vi "NanotecSMCPDDriver.self test.vi"(0 "VISA resource name":refnum<visa-resource-name>, 1 "contollerID":i32=-1, 5 "error in (no error)":errorcluster) -> (14 "VISA resource name out":refnum<visa-resource-name>, 15 "contollerID out":i32=-1, 17 "Self-Test Result Code":i32, 18 "Self-Test Result Message":string, 19 "error out":errorcluster)   [LabVIEW 2014, in "NanotecSMCPDDriver.lvlib"]
doc: "Runs the instrument's self-test routine and returns the test results."
uses:
  NanotecSMCPDDriver.lvlib
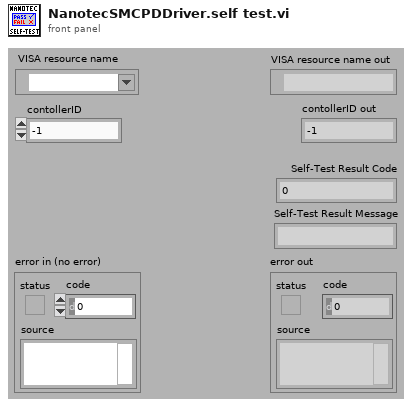
[diagram p1: front panel]
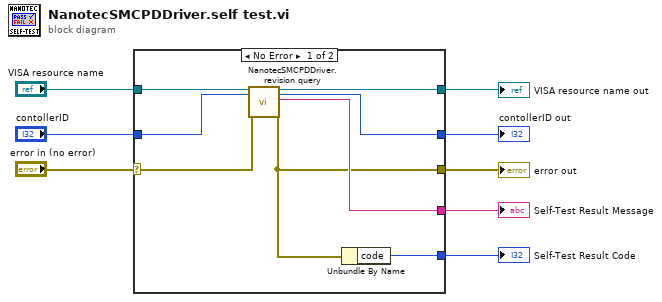
[diagram p0: block diagram]
diagram:
  n1 = case shown="No Error" "error in (no error)" {
    selector: "error in (no error)" -> [w14 w19]
    tunnel: [w10 w19] -> w7
    tunnel: [w12 w18] -> w5
    tunnel: "contollerID" -> [w15 w18]
    tunnel: "VISA resource name" -> [w16 w17]
    tunnel: [w13 w17] -> w3
    tunnel: [w11 _] -> w2
    tunnel: [w9 _] -> w1
    frame No Error {
      n2 = call "NanotecSMCPDDriver.revision query.vi"("VISA resource name"=w16, "contollerID"=w15, "error in (no error)"=w14) -> ("VISA resource name out"=w13:refnum<visa-resource-name>, "contollerID out"=w12:i32, "Instrument Driver Revision"=w11:string, "error out"=w10:errorcluster)  [unwired: 12 in, 1 out]
      n3 = Unbundle By Name(w10) -> ("code"=w9:i32)
    }
    frame Error {
    }
  }
  "Self-Test Result Message" <- w2
  "Self-Test Result Code" <- w1
  "VISA resource name out" <- w3
  "error out" <- w7
  "contollerID out" <- w5
